vi "WSVCAP SHL Host TL Diagnostics Interface.vi"() -> ()   [LabVIEW 2012]
uses:
  Type Defs/WSVCAP SHL Top Level Control Operation Enum.ctl
  Type Defs/WSVCAP SHL Top Level Control Enum.ctl
  <vilib>/rvi/interface/nirviOpenFPGA/nirviOpenFPGA.xnode
  <vilib>/rvi/interface/nirviCloseFPGA/nirviCloseFPGA.xnode
  <vilib>/rvi/interface/nirviMethod/nirviMethod.xnode
  FPGA Bitfiles/WSRFCAPDriver_WiSpryFPGA1_AD7747I2CFPGATLT_3pqPbBuIJ7M.lvbitx
  <vilib>/rvi/errors/niLvFpgaMergeErrorWithErrorCode.vi
  <vilib>/FPGAPlugInAG/PXI-7813R/niLvFpga_Open_PXI-7813R.vi
panel:
  out "SPI Data In":u8[][](array[numeric]) format="%.0x"
  in  "Write/Read SPI":bool
  in  "SPI Data Out":u8[][](array[numeric])=[[0, 0, 0, 0, 0, 0, 0, 0, 0, 0, 0, 0, 0, 0, 0, 0], [0, 0, 0, 0, 0, 0, 0, 0, 0, 0, 0, 0, 0, 0, 0, 0]] format="%.0x"
  out "SPI Data Labels":u8[](array[numeric])=[1, 2, 3, 4, 5, 6, 7, 8, 9, 10, 11, 12, 13, 14, 15, 16]
  in  "SPI Clock Rate (Hz)":dbl=1000000.0
  in  "Read I2C":bool
  in  "Write I2C":bool
  in  "B Data Out":u8[][](array[numeric])=[[0, 0, 0, 0, 0, 0, 0, 0, 0, 0, 0, 0, 0, 0, 0, 0]] format="%.0x"
  in  "A Data Out":u8[][](array[numeric])=[[0, 0, 0, 0, 0, 0, 0, 0, 0, 0, 0, 0, 0, 0, 0, 0]] format="%.0x"
  out "Write Data Labels":u8[](array[numeric])=[1, 2, 3, 4, 5, 6, 7, 8, 9, 10, 11, 12, 13, 14, 15, 16]
  in  "I2C_Sub Address":u8=191 format="%.0x"
  in  "I2C_Slave Address":u8=144 format="%.0x"
  out "B Data In":u8[][](array[numeric]) format="%.0x"
  out "Status":u8[](array[numeric])
  out "A Data In":u8[][](array[numeric]) format="%.0x"
  out "Write Data Labels":u8[](array[numeric])=[1, 2, 3, 4, 5, 6, 7, 8, 9, 10, 11, 12, 13, 14, 15, 16]
  in  "Simulate FPGA":bool
  in  "Error":errorcluster
  in  "Bytes to Read":u8=1
  in  "I2CClock Rate (Hz)":dbl=100000.0
  in  "Exit":bool
  # "Control and Status"
  # "Configure I2C"
  # "Write I2C"
  # "Read I2C"
  # "Configure SPI"
  # "SPI"
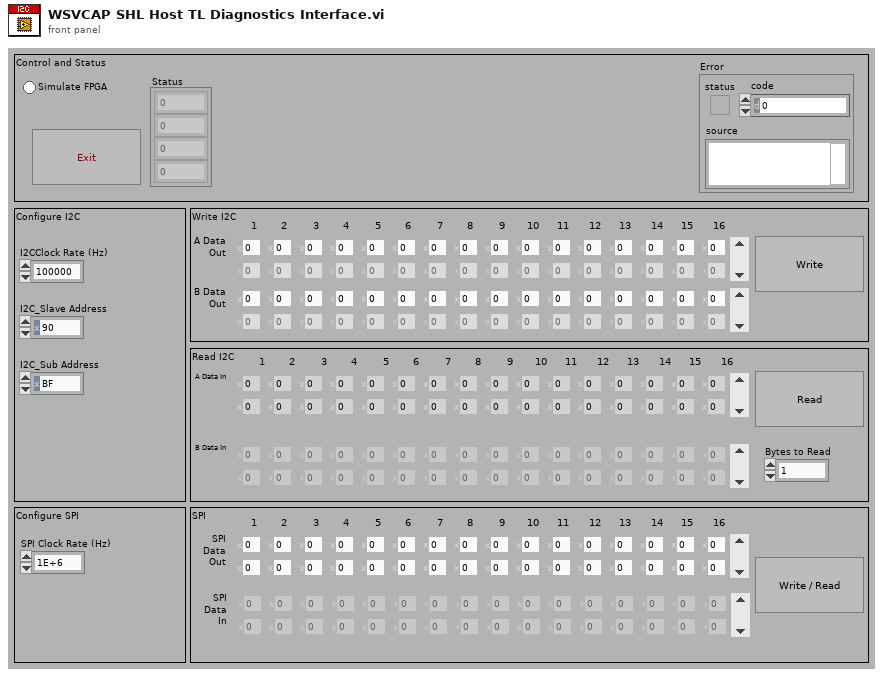
[diagram p1: front panel]
types:
  T1 = typedef "WSVCAP SHL Top Level Control Operation Enum.ctl" = enum16{"Initialize", "Set Control", "Read Control", "Close"}
  T2 = typedef "WSVCAP SHL Top Level Control Enum.ctl" = enum16{"Start", "Cmd", "Transaction", "Wait Ticks", "Socket Mask", "I2C_Slave Address", "I2C_Sub Address", "Bytes to Write", "Bytes to Read", "Write Data", "Write Flag", "Read Data", "Read Flag", "Ack Read", "Read Status Flag", "Ack Read Status", "Status", "Exit"}
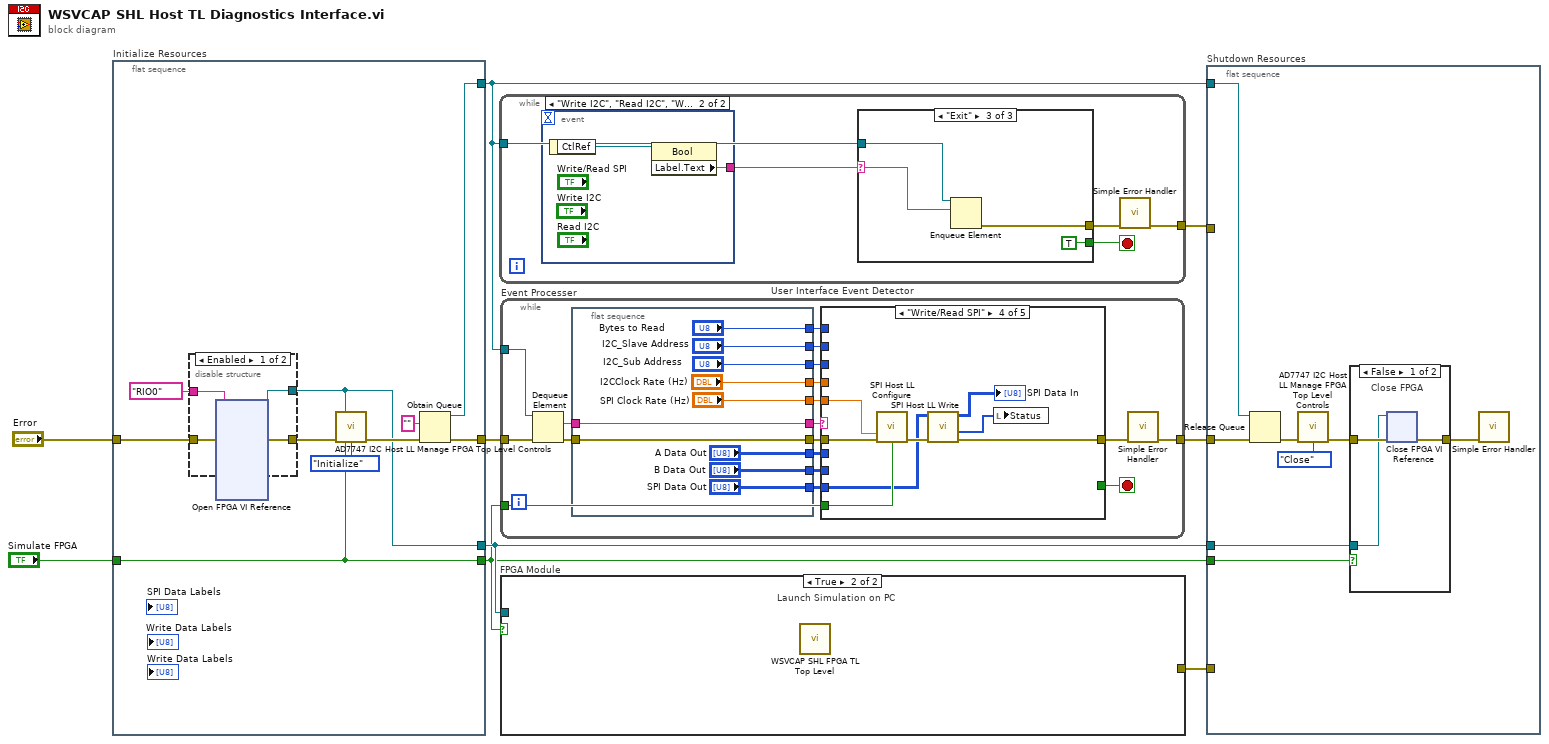
[diagram p0: block diagram]
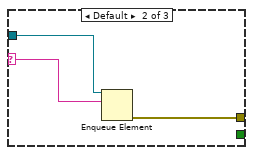
[diagram p5: hidden frame]
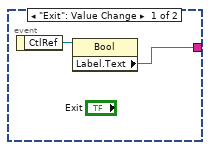
[diagram p6: hidden frame]
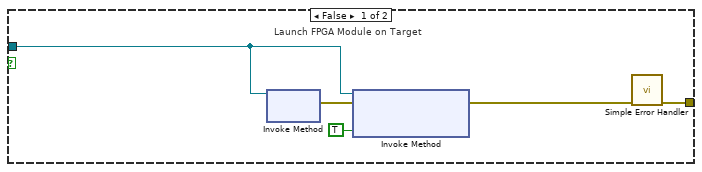
[diagram p7: hidden frame]
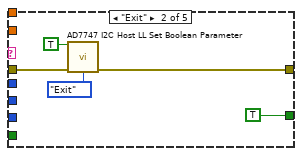
[diagram p9: hidden frame]
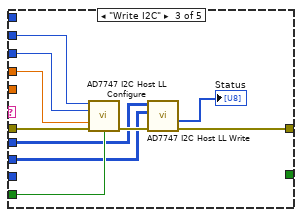
[diagram p10: hidden frame]
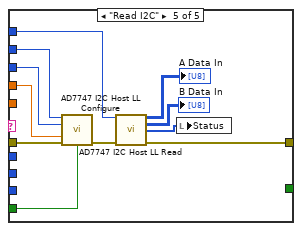
[diagram p11: hidden frame]
diagram:
  n1 = flat-sequence "Initialize Resources" {
    tunnel: "Error" -> [w14]
    tunnel: [w18] -> w8
    tunnel: [w16] -> w7
    tunnel: [w11] -> w1
    tunnel: "Simulate FPGA" -> [w11]
    tunnel: [w10] -> w2
    frame #0 {
      n2 = disable-structure shown="Enabled" {
        disable-tunnel: w14 -> [w23 w24]
        disable-tunnel: [w22 w24] -> w13
        disable-tunnel: [w21 _] -> w10
        disable-tunnel: tag "RIO0" ("resource name") -> [w20 _]
        frame Enabled {
          n3 = xnode "Open FPGA VI Reference"("error in"=w23, "resource name"=w20) -> ("FPGA VI Reference Out"=w21:refnum<k20>, "error out"=w22:errorcluster)
        }
        frame Disabled {
        }
      }
      n4 = call "AD7747 I2C Host LL Manage FPGA Top Level Controls.vi"("FPGA VI Reference (Init Only)"=w10, "error in (no error)"=w13, "Simulate FPGA (Init Only)"=w11, "Operation"=WSVCAP_SHL_Top_Level_Control_Operation_Enum."Initialize") -> ("error out"=w19:errorcluster)  [unwired: 10 in, 1 out]
      n5 = Obtain Queue(element data type="" ("name (unnamed)"), error in (no error)=w19) -> (queue out=w16:refnum<queue>, error out=w18:errorcluster)  [unwired: 3 in, 1 out]
    }
  }
  n6 = while "User Interface Event Detector" {
    tunnel: w7 -> [w28]
    tunnel: [w25] -> w5
    stop <- w26 stop-if-true
    n7 = event shown="[1] \"Write I2C\", \"Read I2C\", \"Write/Read SPI\": Value Change" {
      selector: _ -> [_ _]
      dyn-events: _ -> [_ _]
      timeout: _ -> [_ _]
      tunnel: [w37 w39] -> w29
      event "Exit": Value Change {
        n8 = event-data() -> ("CtlRef"=w38:refnum<vi>)  [unwired: 1 in]
        n9 = property class="Bool"(reference=w38) -> ("Label.Text"=w37:string)  [unwired: 1 in, 2 out]
      }
      event "Write I2C", "Read I2C", "Write/Read SPI": Value Change {
        n10 = event-data() -> ("CtlRef"=w40:refnum<vi>)  [unwired: 1 in]
        n11 = property class="Bool"(reference=w40) -> ("Label.Text"=w39:string)  [unwired: 1 in, 2 out]
      }
    }
    n12 = case shown="\"Exit\"" w29 {
      selector: w29 -> [_ w32 w36]
      tunnel: w28 -> [_ w31 w35]
      tunnel: [_ w30 w34] -> w27
      tunnel: [_ _ TRUE] -> w26
      frame "" {
      }
      frame Default {
        n13 = Enqueue Element(queue=w31, element=w32) -> (error out=w30:errorcluster)  [unwired: 2 in, 2 out]
      }
      frame "Exit" {
        n14 = Enqueue Element(queue=w35, element=w36) -> (error out=w34:errorcluster)  [unwired: 2 in, 2 out]
      }
    }
    n15 = call <vilib>:"Simple Error Handler.vi"("error in (no error)"=w27) -> ("error out"=w25:errorcluster)  [unwired: 4 in, 4 out]
  }
  n16 = while "Event Processer" {
    tunnel: w8 -> [w58]
    tunnel: w7 -> [w57]
    tunnel: [w54] -> w6
    tunnel: w1 -> [w53]
    stop <- w56 stop-if-true
    n17 = Dequeue Element(queue=w57, error in (no error)=w58) -> (element=w50:string, error out=w48:errorcluster)  [unwired: 1 in, 2 out]
    n18 = flat-sequence {
      tunnel: ["I2CClock Rate (Hz)"] -> w52
      tunnel: ["B Data Out"] -> w51
      tunnel: [w67] -> w49
      tunnel: w50 -> [w67]
      tunnel: [w66] -> w47
      tunnel: w48 -> [w66]
      tunnel: ["Bytes to Read"] -> w46
      tunnel: ["I2C_Slave Address"] -> w45
      tunnel: ["I2C_Sub Address"] -> w44
      tunnel: ["A Data Out"] -> w43
      tunnel: ["SPI Clock Rate (Hz)"] -> w42
      tunnel: ["SPI Data Out"] -> w41
      frame #0 {
      }
    }
    n19 = case shown="\"Write/Read SPI\"" w49 {
      tunnel: w47 -> [w69 w71 w83 w91 w102]
      tunnel: [w69 w70 w84 w92 w103] -> w55
      tunnel: [_ TRUE _ _ _] -> w56
      tunnel: w53 -> [_ _ w81 w89 w100]
      tunnel: w52 -> [_ _ w79 _ w96]
      tunnel: w51 -> [_ _ w75 _ _]
      tunnel: w46 -> [_ _ _ _ w97]
      tunnel: w45 -> [_ _ w78 _ w94]
      tunnel: w44 -> [_ _ w77 _ w93]
      tunnel: w43 -> [_ _ w76 _ _]
      tunnel: w42 -> [_ _ _ w85 _]
      tunnel: w41 -> [_ _ _ w88 _]
      frame Default {
      }
      frame "Exit" {
        n20 = call "AD7747 I2C Host LL Set Boolean Parameter.vi"("Boolean In"=TRUE ("Start"), "error in (no error)"=w71, "FPGA Top Level Control"=WSVCAP_SHL_Top_Level_Control_Enum."Exit") -> ("error out"=w70:errorcluster)  [unwired: 12 in]
      }
      frame "Write I2C" {
        n21 = call "AD7747 I2C Host LL Configure.vi"("I2C_Slave Address"=w78, 5:w77, "Clock Rate (Hz)"=w79, "error in"=w83, "Simulate FPGA"=w81) -> ("error out"=w82:errorcluster)  [unwired: 9 in, 1 out]
        n22 = call "AD7747 I2C Host LL Write.vi"("error in"=w82, "B Data Out"=w75, "A Data Out"=w76) -> ("error out"=w84:errorcluster, "Status"=→"Status":u8[])  [unwired: 3 in, 4 out]
      }
      frame "Write/Read SPI" {
        n23 = call "SPI Host LL Configure.vi"("Clock Rate (Hz)"=w85, "error in"=w91, "Simulate FPGA"=w89) -> ("error out"=w90:errorcluster)  [unwired: 11 in, 1 out]
        n24 = call "SPI Host LL Write.vi"("error in"=w90, "SPI Data Out"=w88) -> ("error out"=w92:errorcluster, "Status"=w87:u8[], "SPI Read Data"=→"SPI Data In":u8[][])  [unwired: 7 in]
        n25 = local write "Status"(w87) -> ()
      }
      frame "Read I2C" {
        n26 = call "AD7747 I2C Host LL Configure.vi"("I2C_Slave Address"=w94, 5:w93, "Clock Rate (Hz)"=w96, "error in"=w102, "Simulate FPGA"=w100) -> ("error out"=w101:errorcluster)  [unwired: 9 in, 1 out]
        n27 = call "AD7747 I2C Host LL Read.vi"("Bytes to Read"=w97, "error in"=w101) -> ("A1-A16 Read Data"=→"A Data In":u8[][], "B1-B16 Read Data"=→"B Data In":u8[][], "Status"=w95:u32[], "error out"=w103:errorcluster)  [unwired: 10 in]
        n28 = local write "Status"(w95) -> ()
      }
    }
    n29 = call <vilib>:"Simple Error Handler.vi"("error in (no error)"=w55) -> ("error out"=w54:errorcluster)  [unwired: 4 in, 4 out]
  }
  n30 = case "FPGA Module" shown="True" w1 {
    tunnel: [w108 _] -> w3
    tunnel: w2 -> [w105 _]
    frame False {
      # "Launch FPGA Module on Target"
      n31 = xnode "Invoke Method"("FPGA VI Reference In"=w105) -> ("error out"=w107:errorcluster)  [unwired: 1 in, 1 out]
      n32 = xnode "Invoke Method"("FPGA VI Reference In"=w105, "error in"=w107, "Wait Until Done (F)"=TRUE) -> ("error out"=w104:errorcluster)  [unwired: 1 out]
      n33 = call <vilib>:"Simple Error Handler.vi"("error in (no error)"=w104) -> ("error out"=w108:errorcluster)  [unwired: 4 in, 4 out]
    }
    frame True {
      # "Launch Simulation on PC"
      n34 = call "WSVCAP SHL FPGA TL Top Level.vi"() -> ()  [unwired: 1 in]
    }
  }
  n35 = flat-sequence "Shutdown Resources" {
    tunnel: w7 -> [w116]
    tunnel: w6 -> [w114]
    tunnel: w5 -> [_]
    tunnel: w3 -> [_]
    tunnel: w2 -> [w111]
    tunnel: w1 -> [w109]
    frame #0 {
      n36 = Release Queue(queue=w116, error in (no error)=w114) -> (error out=w113:errorcluster)  [unwired: 1 in, 2 out]
      n37 = call "AD7747 I2C Host LL Manage FPGA Top Level Controls.vi"("error in (no error)"=w113, "Operation"=WSVCAP_SHL_Top_Level_Control_Operation_Enum."Close") -> ("error out"=w112:errorcluster)  [unwired: 12 in, 1 out]
      n38 = case shown="False" w109 {
        tunnel: w112 -> [w119 w120]
        tunnel: w111 -> [w118 _]
        tunnel: [w117 w120] -> w110
        frame False {
          # "Close FPGA"
          n39 = xnode "Close FPGA VI Reference"("FPGA VI Reference In"=w118, "error in"=w119) -> ("error out"=w117:errorcluster)
        }
        frame True {
        }
      }
      n40 = call <vilib>:"Simple Error Handler.vi"("error in (no error)"=w110) -> ()  [unwired: 4 in, 5 out]
    }
  }
